vi "Create_upload_jlink_file.vi"(0 ".mot file":path, 7 "path":path, 9 "Password":string, 11 "error in":errorcluster) -> (15 "error out":errorcluster)   [LabVIEW 2023]
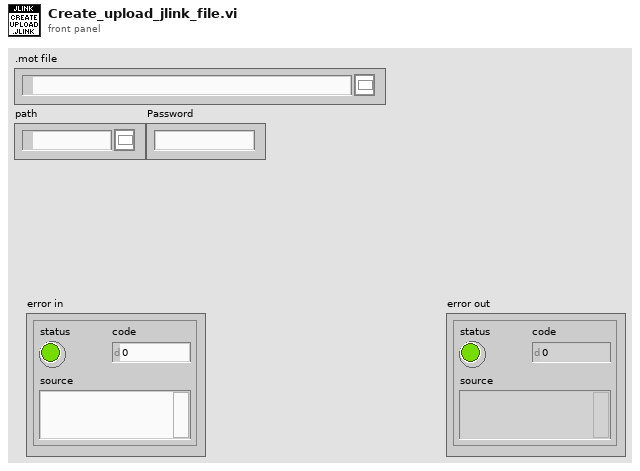
[diagram p1: front panel]
types:
  T1 = enum16{"open", "replace", "create", "open or create", "replace or create", "replace or create with confirmation"}
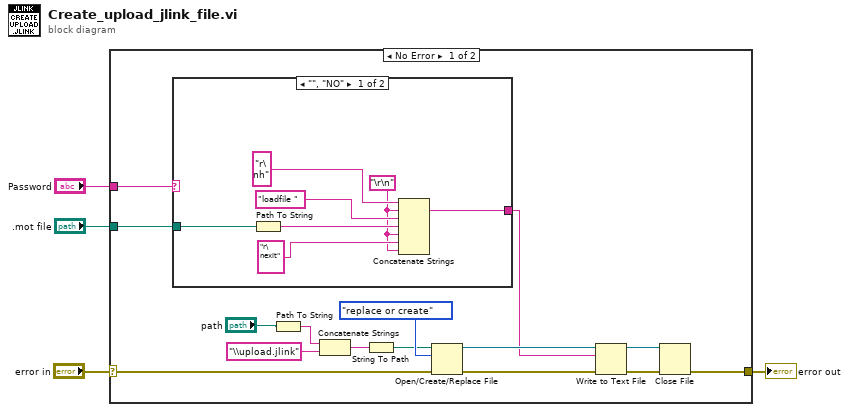
[diagram p0: block diagram]
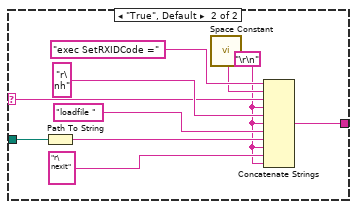
[diagram p2: hidden frame]
diagram:
  n1 = case shown="No Error" "error in" {
    selector: "error in" -> [w9 w37]
    tunnel: [w8 w37] -> w3
    tunnel: "Password" -> [w7 _]
    tunnel: ".mot file" -> [w6 _]
    frame No Error {
      n2 = case shown="\"\", \"NO\"" w7 {
        selector: w7 -> [_ w29]
        tunnel: [w21 w32] -> w5
        tunnel: w6 -> [w20 w27]
        frame "", "NO" {
          w22 = "\r\n"
          n3 = Path To String(path=w20) -> (string=w26:string)
          n4 = Concatenate Strings("r\nh" ("string"), w22, "loadfile " ("string"), w26, w22, "r\nexit" ("string"), w22) -> (w21:string)
        }
        frame "True", Default {
          w28 = "\r\n"
          n5 = Path To String(path=w27) -> (string=w36:string)
          n6 = call <vilib>:"Space Constant.vi"() -> ("String"=w30:string)
          n7 = Concatenate Strings("exec SetRXIDCode =", w30, w29, w28, "r\nh" ("string"), w28, "loadfile " ("string"), w36, w28, "r\nexit" ("string"), w28) -> (w32:string)
        }
      }
      n8 = Path To String(path="path") -> (string=w12:string)
      n9 = Concatenate Strings(w12, "\\upload.jlink" ("string")) -> (w13:string)
      n10 = String To Path(string=w13) -> (path=w11:path)
      n11 = Open/Create/Replace File(file path (use dialog)=w11, error in=w9, operation (0:open)=T1."replace or create") -> (refnum out=w18:refnum<file>, error out=w17:errorcluster)  [unwired: 3 in, 1 out]
      n12 = Write to Text File(file (use dialog)=w18, text=w5, error in=w17) -> (refnum out=w16:refnum<file>, error out=w15:errorcluster)  [unwired: 1 in, 1 out]
      n13 = Close File(refnum=w16, error in=w15) -> (error out=w8:errorcluster)  [unwired: 1 out]
    }
    frame Error {
    }
  }
  "error out" <- w3
